vi "Square Root.vi"() -> ()   [LabVIEW 2014]
panel:
  out "Square Root Value":dbl
  in  "Number":dbl
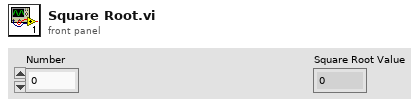
[diagram p1: front panel]
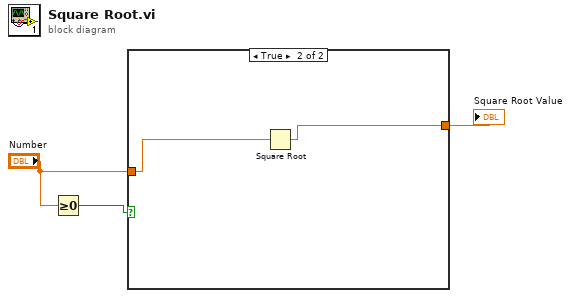
[diagram p0: block diagram]
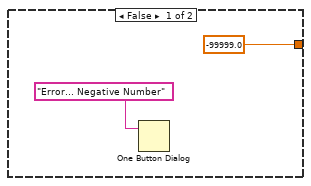
[diagram p2: hidden frame]
diagram:
  n1 = Greater Or Equal To 0?(x="Number") -> (x >= 0?=w3:bool)
  n2 = case shown="True" w3 {
    tunnel: "Number" -> [_ w7]
    tunnel: [-99999.0 ("Square Root Value") w6] -> w1
    frame False {
      n3 = One Button Dialog(message="Error... Negative Number") -> ()  [unwired: 1 in, 1 out]
    }
    frame True {
      n4 = Square Root(x=w7) -> (sqrt(x)=w6:dbl)
    }
  }
  "Square Root Value" <- w1
